vi "Launch Async Action.vi"(8 "error in (no error)":errorcluster, 9 "Message Data":variant, 10 "Message":string, 11 "Async Action In":refnum<class "Async Action.lvclass">) -> (0 "error out":errorcluster, 3 "Async Action Out":refnum<class "Async Action.lvclass">)   [LabVIEW 2020, in "Async Action.lvclass"]
doc: "Launches an asynchronous helper loop. Multiple helper loops may be launched using multiple calls to this VI. The Message and Message Data provided to this VI will be available in the Helper Action.vi once running."
uses:
  Async Action.lvclass
  Process/Process.lvclass
  <vilib>/Utility/error.llb/Error Cluster From Error Code.vi
  <vilib>/ErrorRing/Error Ring.xnode
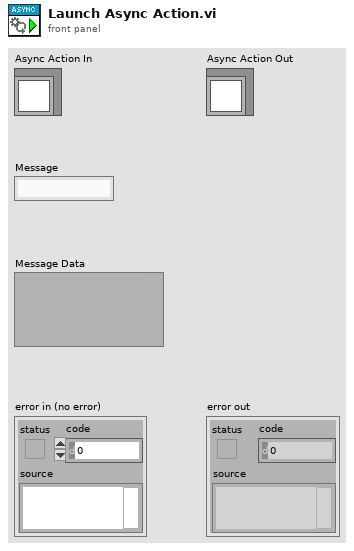
[diagram p1: front panel]
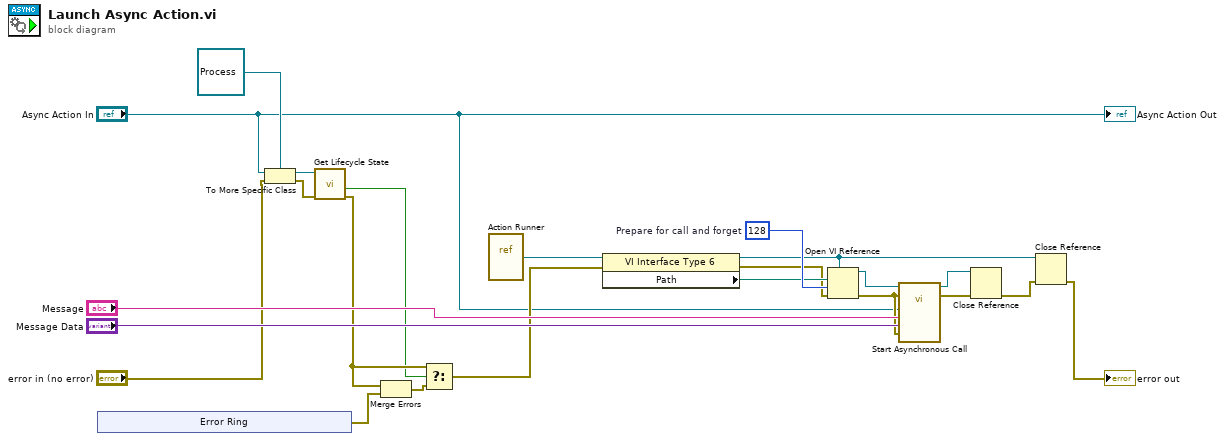
[diagram p0: block diagram]
diagram:
  w17 = 128  # Prepare for call and forget
  n1 = xnode "Error Ring"() -> ("error out"=w5:errorcluster)
  n2 = To More Specific Class(target class=refnum<class "Process.lvclass"> refnum ("Process Out"), reference="Async Action In", error in="error in (no error)") -> (specific class reference=w10:refnum<class "Process.lvclass">, error out=w9:errorcluster)
  n3 = call "Get Lifecycle State.vi"("error in (no error)"=w9, "Process In"=w10) -> ("error out"=w8:errorcluster, "In Process Loop?"=w7:bool)  [unwired: 6 in, 2 out]
  n4 = Merge Errors(w8, w5) -> (w6:errorcluster)
  n5 = Select(t=w8, s=w7, f=w6) -> (s? t:f=w4:errorcluster)
  n6 = vi-ref "Action Runner.vi"() -> (w18:refnum<vi>)
  n7 = property class="VI Interface Type 6"(reference=w18, error in=w4) -> (reference out=w11:refnum<vi>, error out=w13:errorcluster, "Path"=w15:path)
  n8 = Open VI Reference(type specifier VI Refnum (for type only)=w11, vi path=w15, options=w17, error in (no error)=w13) -> (vi reference=w16:refnum<vi>, error out=w14:errorcluster)  [unwired: 2 in]
  n9 = call-by-ref "Start Asynchronous Call"(reference=w16, error in=w14, 8:"error in (no error)"=w14, "Message Data"="Message Data", "Message"="Message", "Asynchronous Action In"="Async Action In") -> (reference out=w20:refnum<vi>, error out=w19:errorcluster)  [unwired: 6 in, 2 out]
  n10 = Close Reference(reference=w20, error in (no error)=w19) -> (error out=w12:errorcluster)
  n11 = Close Reference(reference=w11, error in (no error)=w12) -> (error out=→"error out":errorcluster)
  "Async Action Out" <- "Async Action In"
